vi "apache_master.vi"() -> ()   [LabVIEW 2016]
uses:
  <vilib>/httpClient/LabVIEWHTTPClient.lvlib
  <vilib>/httpClient/POSTBuffer.vi
panel:
  out "Longitude":string
  out "Error":string
  out "Latitude":string
  out "Battery Level":dbl(slide) scale=0.0..100.0
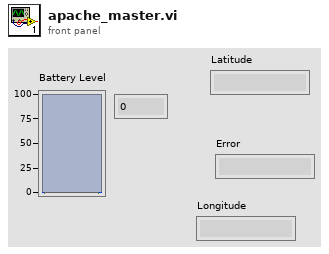
[diagram p1: front panel]
types:
  T1 = typedef "LabVIEWHTTPClient.lvlib/ClientHandle.ctl" = refnum<k1>
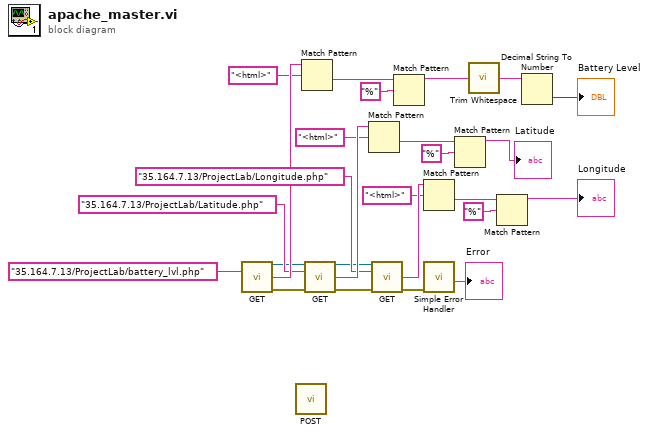
[diagram p0: block diagram]
diagram:
  n1 = call <vilib>:"GET.vi"("url"="35.164.7.13/ProjectLab/battery_lvl.php") -> ("client handle out"=w8:T1, "body"=w25:string, "error out"=w6:errorcluster)  [unwired: 11 in, 1 out]
  n2 = call-poly <vilib>:"POST.vi"() -> ()  [unwired: 12 in, 4 out]
  n3 = Match Pattern(string=w25, regular expression="<html>") -> (after substring=w23:string)  [unwired: 1 in, 3 out]
  n4 = call <vilib>:"GET.vi"("client handle"=w8, "url"="35.164.7.13/ProjectLab/Latitude.php", "error in (no error)"=w6) -> ("client handle out"=w7:T1, "body"=w17:string, "error out"=w5:errorcluster)  [unwired: 9 in, 1 out]
  n5 = Match Pattern(string=w17, regular expression="<html>") -> (after substring=w15:string)  [unwired: 1 in, 3 out]
  n6 = call <vilib>:"GET.vi"("client handle"=w7, "url"="35.164.7.13/ProjectLab/Longitude.php", "error in (no error)"=w5) -> ("body"=w12:string, "error out"=w4:errorcluster)  [unwired: 9 in, 2 out]
  n7 = Match Pattern(string=w23, regular expression="%") -> (before substring=w21:string)  [unwired: 1 in, 3 out]
  n8 = Match Pattern(string=w12, regular expression="<html>") -> (after substring=w10:string)  [unwired: 1 in, 3 out]
  n9 = call <vilib>:"Simple Error Handler.vi"("error in (no error)"=w4) -> ("source out"=→"Error":string)  [unwired: 4 in, 4 out]
  n10 = Match Pattern(string=w15, regular expression="%") -> (before substring=→"Latitude":string)  [unwired: 1 in, 3 out]
  n11 = call <vilib>:"Trim Whitespace.vi"("string"=w21) -> ("trimmed string"=w20:string)  [unwired: 1 in]
  n12 = Match Pattern(string=w10, regular expression="%") -> (before substring=→"Longitude":string)  [unwired: 1 in, 3 out]
  n13 = Decimal String To Number(string=w20) -> (number=→"Battery Level":i32)  [unwired: 2 in, 1 out]
